vi "HTML Project Description Save.vi"(8 "error in (no error)":errorcluster) -> (0 "error out":errorcluster)   [LabVIEW 2014, in "lvprj2html.lvlib"]
uses:
  lvprj2html.lvlib
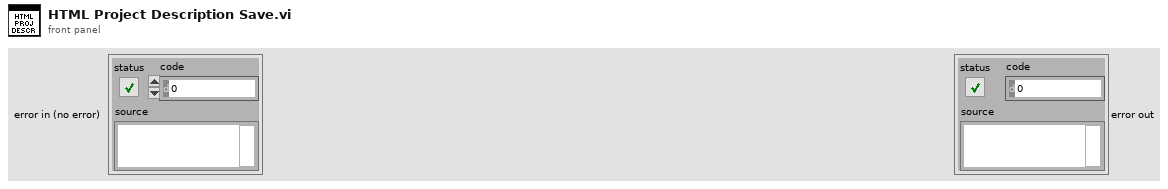
[diagram p1: front panel]
types:
  T1 = enum16{"open", "replace", "create", "open or create", "replace or create", "replace or create with confirmation"}
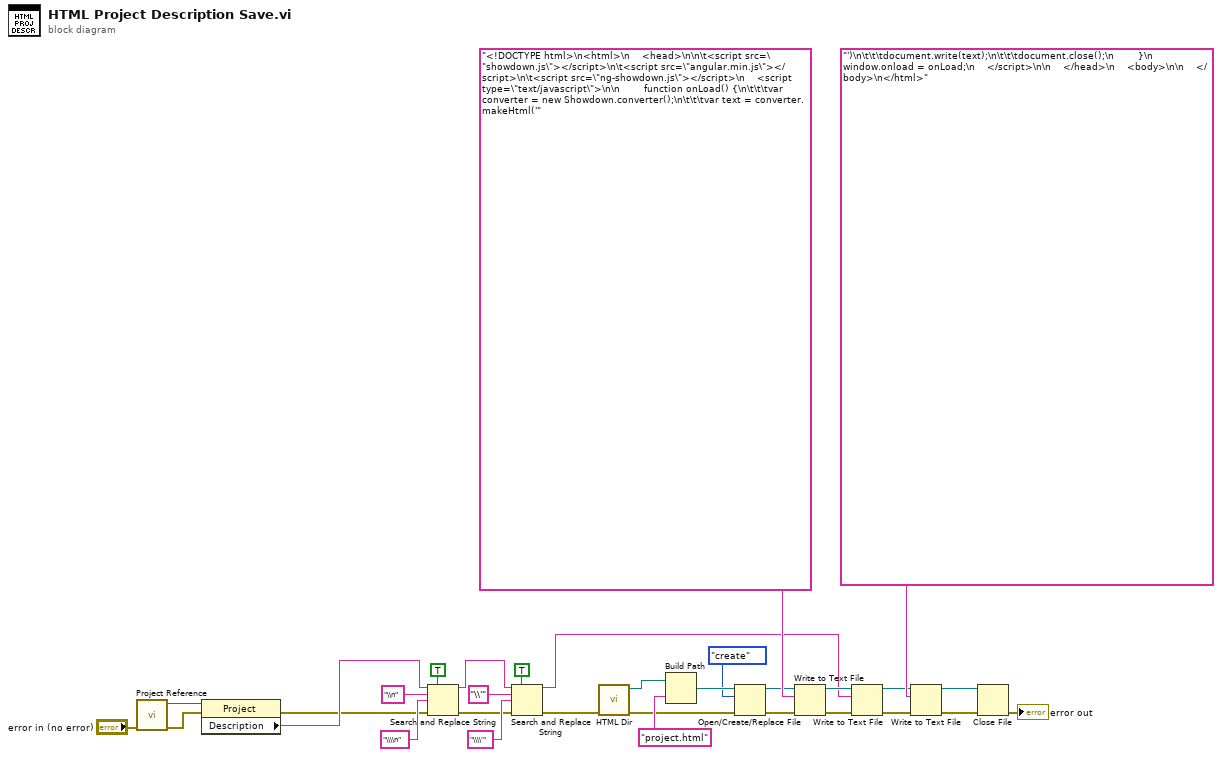
[diagram p0: block diagram]
diagram:
  n1 = call "Project Reference.vi"("error in (no error)"="error in (no error)") -> ("error out"=w9:errorcluster, "prj ref"=w28:refnum<vi>)  [unwired: 9 in]
  n2 = property class="Project"(reference=w28, error in=w9) -> (error out=w11:errorcluster, "Description"=w13:string)  [unwired: 1 out]
  n3 = Search and Replace String(replace all?=TRUE ("replace all? (F)"), input string=w13, search string="\\n", replace string="\\\\n" ("replace string (\"\")"), error in=w11) -> (result string=w14:string, error out=w10:errorcluster)  [unwired: 3 in, 2 out]
  n4 = Search and Replace String(replace all?=TRUE ("replace all? (F)"), input string=w14, search string="\\'", replace string="\\\\'" ("replace string (\"\")"), error in=w10) -> (result string=w12:string, error out=w8:errorcluster)  [unwired: 3 in, 2 out]
  n5 = call "HTML Dir.vi"("error in (no error)"=w8) -> ("error out"=w7:errorcluster, "path"=w26:path)  [unwired: 9 in]
  n6 = Build Path(base path=w26, name or relative path="project.html") -> (appended path=w24:path)
  n7 = Open/Create/Replace File(file path (use dialog)=w24, error in=w7, operation (0:open)=T1."create") -> (refnum out=w22:refnum<file>, error out=w6:errorcluster)  [unwired: 3 in, 1 out]
  n8 = Write to Text File(file (use dialog)=w22, text="<!DOCTYPE html>\n<html>\n    <head>\n\n\t<script src=\"showdown.js\"></script>\n\t<script src=\"angular.min.js\"></script>\n\t<script src=\"ng-showdown.js\"></script>\n    <script type=\"text/javascript\">\n\n        function onLoad() {\n\t\t\tvar converter = new Showdown.converter();\n\t\t\tvar text = converter.makeHtml('", error in=w6) -> (refnum out=w29:refnum<file>, error out=w5:errorcluster)  [unwired: 1 in, 1 out]
  n9 = Write to Text File(file (use dialog)=w29, text=w12, error in=w5) -> (refnum out=w30:refnum<file>, error out=w4:errorcluster)  [unwired: 1 in, 1 out]
  n10 = Write to Text File(file (use dialog)=w30, text="')\n\t\t\tdocument.write(text);\n\t\t\tdocument.close();\n        }\n        window.onload = onLoad;\n    </script>\n\n    </head>\n    <body>\n\n    </body>\n</html>", error in=w4) -> (refnum out=w21:refnum<file>, error out=w3:errorcluster)  [unwired: 1 in, 1 out]
  n11 = Close File(refnum=w21, error in=w3) -> (error out=→"error out":errorcluster)  [unwired: 1 out]
